vi "Pull Info From XNET Database.vi"(8 "error in":errorcluster, 10 "Frame Configuration":T1 {"CRC"."Data Type" items=["Signed", "Unsigned", "IEEE Float"]; "Rolling Counter"."Data Type" items=["Signed", "Unsigned", "IEEE Float"]; "Input Channels"."Data Type" items=["Signed", "Unsigned", "IEEE Float"]}, 11 "Parent Ref":T4=18446744073709551615 format="%.0x") -> (0 "error out":errorcluster, 2 "Frame Configuration":T1 {"CRC"."Data Type" items=["Signed", "Unsigned", "IEEE Float"]; "Rolling Counter"."Data Type" items=["Signed", "Unsigned", "IEEE Float"]; "Input Channels"."Data Type" items=["Signed", "Unsigned", "IEEE Float"]}, 3 "Item Ref out":T4 format="%.0x")   [LabVIEW 2016, in "LIN Frame Protection Addon System Explorer.lvlib"]
uses:
  LIN Frame Protection Addon System Explorer.lvlib
  Shared/Types/FrameConfiguration.ctl
  Shared/Types/InputChannelConfiguration.ctl
  Shared/Types/Protection Type.ctl
  <vilib>/NI Veristand/Custom Device API/Custom Device Item Ref.ctl
  NationalInstruments.VeriStand.SystemStorage
  NationalInstruments.VeriStand
  <vilib>/NI Veristand/Custom Device API/Custom Device API.lvlib
  <vilib>/NI Veristand/Custom Device Tools/Custom Device Utility Library/Custom Device Utility Library.lvlib
  <resource>/objmgr/xnet.rc
  Shared/LIN Frame Protection Addon Shared.lvlib
panel:
  out "Value":string
  out "Array":string[](array[string])
  out "CycleTime":dbl
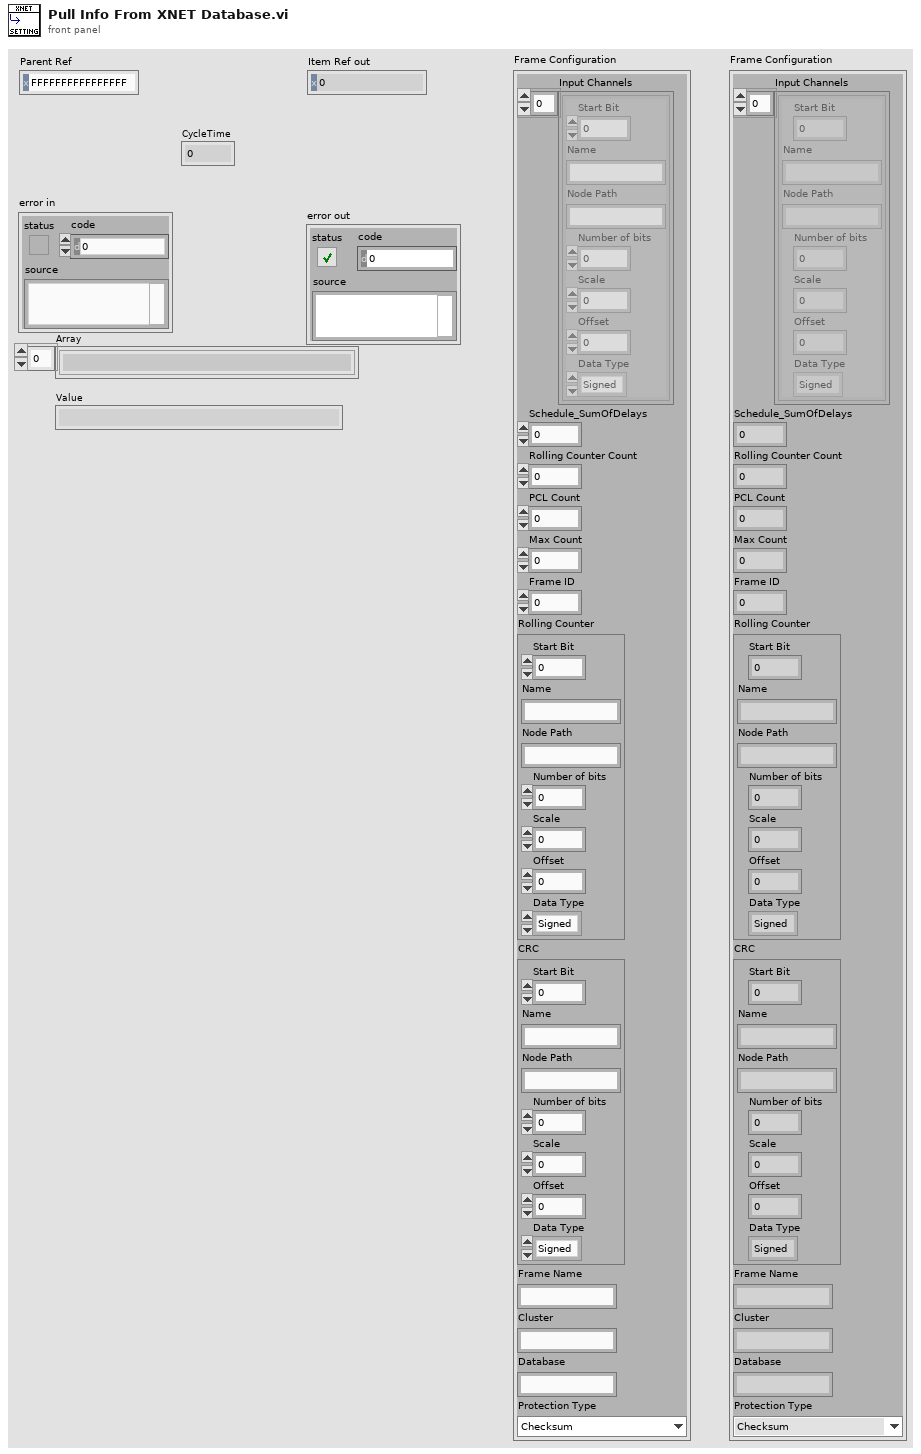
[diagram p1: front panel]
types:
  T1 = typedef "LIN Frame Protection Addon Shared.lvlib/FrameConfiguration.ctl" = cluster{"Input Channels":T2[], "Schedule_SumOfDelays":dbl, "Rolling Counter Count":dbl, "PCL Count":u64, "Max Count":dbl, "Frame ID":u32, "Rolling Counter":T2, "CRC":T2, "Frame Name":string, "Cluster":string, "Database":string, "Protection Type":T3}
  T2 = typedef "LIN Frame Protection Addon Shared.lvlib/InputChannelConfiguration.ctl" = cluster{"Start Bit":i32, "Name":string, "Node Path":string, "Number of bits":i32, "Scale":dbl, "Offset":dbl, "Data Type":u32}
  T3 = typedef "LIN Frame Protection Addon Shared.lvlib/Protection Type.ctl" = enum16{"Checksum", "CRC", "None (Counter Only)"}
  T4 = typedef "Custom Device API.lvlib/Custom Device Item Ref.ctl" = u64
  T5 = typedef "Custom Device API.lvlib/Custom Device Pointer.ctl" = refnum<k24>
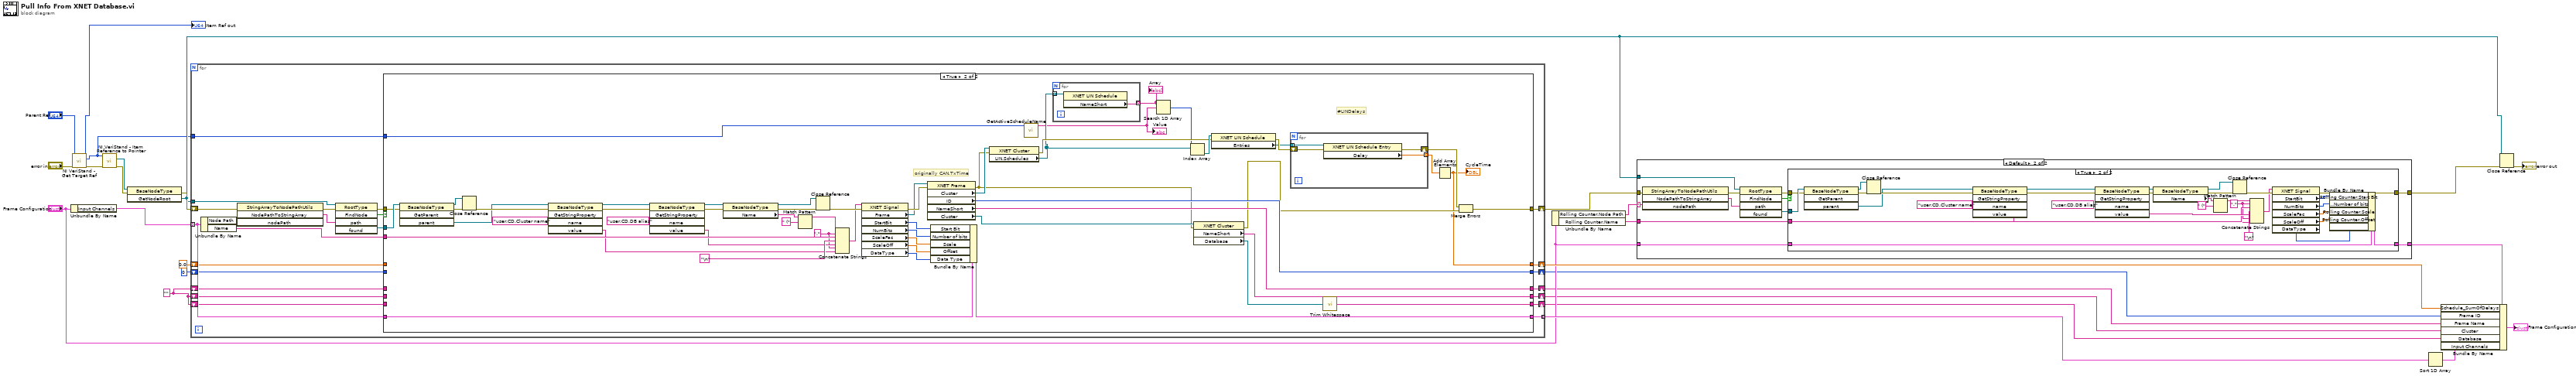
[diagram p0: block diagram]
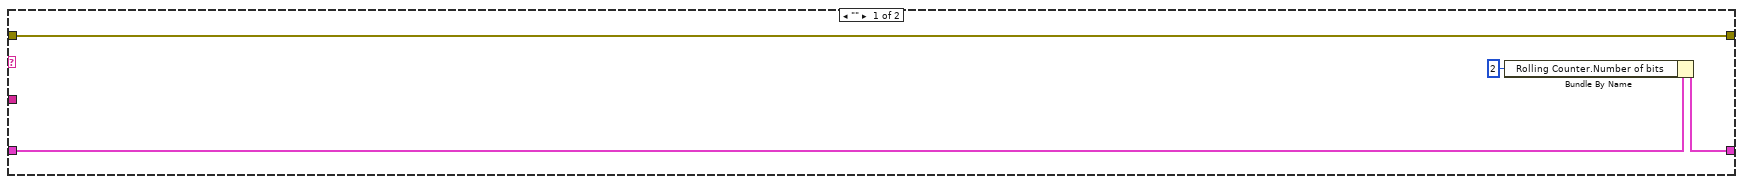
[diagram p2: hidden frame]
diagram:
  w5 = "" ("NameShort")
  n1 = Unbundle By Name("Frame Configuration") -> ("Input Channels"=w25:T2[])
  n2 = call <vilib>:"NI VeriStand - Get Target Ref.vi"("error in"="error in", "Item Ref in"="Parent Ref") -> ("error out"=w26:errorcluster, "Target Ref"=w1:T4, "Item Ref out"=→"Item Ref out":T4)  [unwired: 6 in, 1 out]
  n3 = call <vilib>:"NI VeriStand - Item Reference to Pointer.vi"("error in (no error)"=w26, "Item Ref in"=w1) -> ("error out"=w21:errorcluster, "Node Pointer"=w22:T5)  [unwired: 6 in, 2 out]
  n4 = invoke class="BaseNodeType" method="GetNodeRoot"(reference=w22, error in=w21) -> (error out=w20:errorcluster, "GetNodeRoot"=w13:refnum<k24>)  [unwired: 1 in, 1 out]
  n5 = for {
    tunnel: w13 -> [w45]
    shift-right: [w47] -> w12
    shift-left: w20 -> [w51]
    tunnel: w25 -> [w41] mode=indexing
    tunnel: [w40] -> w19 mode=indexing
    shift-right: [w39] -> w15
    shift-left: 0.0 ("CAN.TxTime") -> [w38]
    shift-right: [w37] -> w6
    shift-left: u32 0 ("ID") -> [w36]
    shift-right: [w35] -> w2
    shift-left: w5 -> [w34]
    shift-right: [w33] -> w3
    shift-left: w5 -> [w31]
    shift-right: [w32] -> w4
    shift-left: w5 -> [w30]
    tunnel: w1 -> [w29]
    n6 = Unbundle By Name(w41) -> ("Node Path"=w46:string, "Name"=w42:string)
    n7 = invoke class="StringArrayToNodePathUtils" method="NodePathToStringArray"(error in=w51, "nodePath"=w46) -> (error out=w50:errorcluster, "NodePathToStringArray"=w44:string[])  [unwired: 2 in, 2 out]
    n8 = invoke class="RootType" method="FindNode"(reference=w45, error in=w50, "path"=w44) -> (error out=w43:errorcluster, "FindNode"=w48:bool, "found"=w49:refnum<k24>)  [unwired: 2 in, 2 out]
    n9 = case shown="True" w48 {
      tunnel: w43 -> [w58 w112]
      tunnel: w49 -> [_ w113]
      tunnel: [w58 w68] -> w47
      tunnel: w42 -> [_ w110]
      tunnel: w41 -> [w57 w109]
      tunnel: [w57 w105] -> w40
      tunnel: [w56 w65] -> w39
      tunnel: w38 -> [w56 _]
      tunnel: [w55 w93] -> w37
      tunnel: w36 -> [w55 _]
      tunnel: [w54 w92] -> w35
      tunnel: w34 -> [w54 _]
      tunnel: [w53 w90] -> w33
      tunnel: [w52 w88] -> w32
      tunnel: w31 -> [w53 _]
      tunnel: w30 -> [w52 _]
      tunnel: w29 -> [_ w63]
      frame False {
      }
      frame True {
        w77 = "." ("string")
        # "#LINDelays"
        # "originally CAN.TxTime"
        n10 = invoke class="BaseNodeType" method="GetParent"(reference=w113, error in=w112) -> (reference out=w100:refnum<k24>, error out=w101:errorcluster, "parent"=w80:refnum<k24>)  [unwired: 2 in, 1 out]
        n11 = Close Reference(reference=w100, error in (no error)=w101) -> (error out=w82:errorcluster)
        n12 = invoke class="BaseNodeType" method="GetStringProperty"(reference=w80, error in=w82, "name"="user.CD.Cluster name") -> (reference out=w79:refnum<k24>, error out=w81:errorcluster, "value"=w76:string)  [unwired: 2 in, 2 out]
        n13 = invoke class="BaseNodeType" method="GetStringProperty"(reference=w79, error in=w81, "name"="user.CD.DB alias") -> (reference out=w84:refnum<k24>, error out=w98:errorcluster, "value"=w78:string)  [unwired: 2 in, 2 out]
        n14 = property class="BaseNodeType"(reference=w84, error in=w98) -> (reference out=w99:refnum<k24>, error out=w97:errorcluster, "Name"=w96:string)
        n15 = Match Pattern(string=w96, regular expression=" (") -> (before substring=w87:string)  [unwired: 1 in, 3 out]
        n16 = Close Reference(reference=w99, error in (no error)=w97) -> (error out=w102:errorcluster)
        n17 = Concatenate Strings(w87, w77, w110, "\n", w78, w77, w76) -> (w75:string)
        n18 = property class="XNET Signal"(reference=w75, error in=w102) -> (error out=w103:errorcluster, "Frame"=w85:refnum<k21>, "StartBit"=w104:u32, "NumBits"=w108:u32, "ScaleFac"=w106:dbl, "ScaleOff"=w107:dbl, "DataType"=w94:u32)  [unwired: 1 out]
        n19 = property class="XNET Frame"(reference=w85, error in=w103) -> (error out=w70:errorcluster, "Cluster"=w74:refnum<k21>, "ID"=w93:u32, "NameShort"=w92:string, "Cluster"=w91:refnum<k21>)  [unwired: 1 out]
        n20 = Bundle By Name(cluster=w109, "Start Bit"=w104, "Number of bits"=w108, "Scale"=w106, "Offset"=w107, "Data Type"=w94) -> (w105:T2)
        n21 = property class="XNET Cluster"(reference=w74, error in=w70) -> (error out=w69:errorcluster, "LIN.Schedules"=w62:refnum<k21>[])  [unwired: 1 out]
        n22 = call "GetActiveScheduleName.vi"("Target Ref"=w63) -> ("Value"=w60:string)  [unwired: 10 in]
        "Value" <- w60
        n23 = for {
          tunnel: [w115] -> w61 mode=indexing
          tunnel: w62 -> [w114] mode=indexing
          n24 = property class="XNET LIN Schedule"(reference=w114) -> ("NameShort"=w115:string)  [unwired: 1 in, 2 out]
        }
        "Array" <- w61
        n25 = Search 1D Array(1D array=w61, element=w60) -> (index of element=w59:i32)  [unwired: 1 in]
        n26 = Index Array(array=w62, index=w59) -> (element=w73:refnum<k21>)
        n27 = property class="XNET Cluster"(reference=w91, error in=w70) -> (error out=w67:errorcluster, "NameShort"=w90:string, "Database"=w89:refnum<k21>)  [unwired: 1 out]
        n28 = property class="XNET LIN Schedule"(reference=w73, error in=w69) -> (error out=w72:errorcluster, "Entries"=w71:refnum<k21>[])  [unwired: 1 out]
        n29 = for {
          tunnel: w71 -> [w116] mode=indexing
          tunnel: [w118] -> w64 mode=indexing
          shift-right: [w117] -> w66
          shift-left: w72 -> [w119]
          n30 = property class="XNET LIN Schedule Entry"(reference=w116, error in=w119) -> (error out=w117:errorcluster, "Delay"=w118:dbl)  [unwired: 1 out]
        }
        n31 = call <vilib>:"Trim Whitespace.vi"("string"=w89) -> ("trimmed string"=w88:string)  [unwired: 1 in]
        n32 = Add Array Elements(numeric array=w64) -> (sum=w65:dbl)
        "CycleTime" <- w65
        n33 = Merge Errors(w66, w67) -> (w68:errorcluster)
      }
    }
  }
  n34 = Unbundle By Name("Frame Configuration") -> ("Rolling Counter.Node Path"=w8:string, "Rolling Counter.Name"=w14:string)
  n35 = case shown="Default" w8 {
    selector: w8 -> [_ w124]
    tunnel: w14 -> [_ w130]
    tunnel: w13 -> [_ w129]
    tunnel: w12 -> [w123 w128]
    tunnel: [w123 w127] -> w11
    tunnel: "Frame Configuration" -> [w122 w126]
    tunnel: [w121 w125] -> w9
    frame "" {
      n36 = Bundle By Name(cluster=w122, "Rolling Counter.Number of bits"=u32 2 ("Rolling Counter Length")) -> (w121:T1)
    }
    frame Default {
      n37 = invoke class="StringArrayToNodePathUtils" method="NodePathToStringArray"(error in=w128, "nodePath"=w124) -> (error out=w135:errorcluster, "NodePathToStringArray"=w132:string[])  [unwired: 2 in, 2 out]
      n38 = invoke class="RootType" method="FindNode"(reference=w129, error in=w135, "path"=w132) -> (error out=w131:errorcluster, "FindNode"=w133:bool, "found"=w134:refnum<k24>)  [unwired: 2 in, 2 out]
      n39 = case shown="True" w133 {
        tunnel: w131 -> [w137 w168]
        tunnel: w134 -> [_ w169]
        tunnel: [w137 w157] -> w127
        tunnel: w130 -> [_ w164]
        tunnel: w126 -> [w136 w163]
        tunnel: [w136 w161] -> w125
        frame False {
        }
        frame True {
          w140 = "." ("string")
          n40 = invoke class="BaseNodeType" method="GetParent"(reference=w169, error in=w168) -> (reference out=w158:refnum<k24>, error out=w159:errorcluster, "parent"=w142:refnum<k24>)  [unwired: 2 in, 1 out]
          n41 = Close Reference(reference=w158, error in (no error)=w159) -> (error out=w144:errorcluster)
          n42 = invoke class="BaseNodeType" method="GetStringProperty"(reference=w142, error in=w144, "name"="user.CD.Cluster name") -> (reference out=w141:refnum<k24>, error out=w143:errorcluster, "value"=w139:string)  [unwired: 2 in, 2 out]
          n43 = invoke class="BaseNodeType" method="GetStringProperty"(reference=w141, error in=w143, "name"="user.CD.DB alias") -> (reference out=w154:refnum<k24>, error out=w156:errorcluster, "value"=w165:string)  [unwired: 2 in, 2 out]
          n44 = property class="BaseNodeType"(reference=w154, error in=w156) -> (reference out=w153:refnum<k24>, error out=w155:errorcluster, "Name"=w151:string)
          n45 = Match Pattern(string=w151, regular expression=" (") -> (before substring=w150:string)  [unwired: 1 in, 3 out]
          n46 = Close Reference(reference=w153, error in (no error)=w155) -> (error out=w160:errorcluster)
          n47 = Concatenate Strings(w150, w140, w164, "\n", w165, w140, w139) -> (w138:string)
          n48 = property class="XNET Signal"(reference=w138, error in=w160) -> (error out=w157:errorcluster, "StartBit"=w162:u32, "NumBits"=w149:u32, "ScaleFac"=w148:dbl, "ScaleOff"=w147:dbl, "DataType"=w146:u32)  [unwired: 1 out]
          n49 = Bundle By Name(cluster=w163, "Rolling Counter.Start Bit"=w162, "Rolling Counter.Number of bits"=w149, "Rolling Counter.Scale"=w148, "Rolling Counter.Offset"=w147, "Rolling Counter.Data Type"=w146) -> (w161:T1)
        }
      }
    }
  }
  n50 = Sort 1D Array(array=w19) -> (sorted array=w17:T2[])
  n51 = Bundle By Name(cluster=w9, "Schedule_SumOfDelays"=w15, "Frame ID"=w6, "Frame Name"=w2, "Cluster"=w3, "Database"=w4, "Input Channels"=w17) -> (→"Frame Configuration":T1)
  n52 = Close Reference(reference=w13, error in (no error)=w11) -> (error out=→"error out":errorcluster)
